vi "Destroy.vi"(8 "error in (no error)":errorcluster, 11 "Result Model in":refnum<class "Result Model.lvclass">) -> (0 "error out":errorcluster)   [LabVIEW 2020, in "Result Model.lvclass"]
uses:
  Result Model.lvclass
  Result Model.lvclass/Result Model.ctl
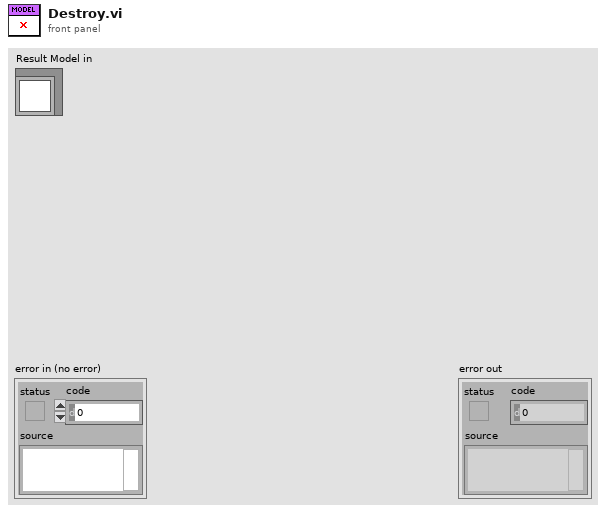
[diagram p1: front panel]
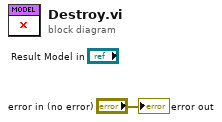
[diagram p0: block diagram]
diagram:
  "error out" <- "error in (no error)"
